vi "Test DUT Self Test Triggers Status Broadcast Message if Not Powered.vi"(8 "error in (no error)":errorcluster, 11 "Device Under Test Test In":refnum<class "Device Under Test Test.lvclass">) -> (0 "error out":errorcluster, 3 "Device Under Test Test Out":refnum<class "Device Under Test Test.lvclass">)   [LabVIEW 2020, in "Device Under Test Test.lvclass"]
uses:
  Device Under Test Test.lvclass
  C:/Program Files (x86)/National Instruments/LabVIEW 2020/vi.lib/Astemes/LUnit/Test Case.lvclass
  Device Under Test/Device Under Test.lvclass
  C:/Program Files (x86)/National Instruments/LabVIEW 2020/vi.lib/Astemes/Triarc Framework/Process/Process.lvclass
  <vilib>/Astemes/Triarc Framework/Process/Process.lvclass/Process.ctl
  <vilib>/Astemes/LUnit/Test Case.lvclass/Test Case.ctl
  <vilib>/Astemes/Triarc Framework/Broadcast Event Helpers/Execution timer.vi
  <vilib>/Astemes/Triarc Framework/Process/Private/SubVIs/Wait for finish.vi
  <vilib>/Astemes/Triarc Framework/Process/Private/SubVIs/Set Lifecycle State.vi
  <vilib>/Astemes/Triarc Framework/Process/Protected/Messaging/Send Message.vi
  <vilib>/Astemes/LUnit/Core/LUnit Test Case/Private/Append Pass Result.vi
  <vilib>/Astemes/LUnit/Core/LUnit Test Case/Private/Append Fail Result.vi
  <vilib>/Astemes/Triarc Framework/Process/Private/SubVIs/Handle Debug Data.vi
  <vilib>/Astemes/LUnit/Core/LUnit Test Case/Private/Run In UI.vi
  <vilib>/Utility/error.llb/Clear Errors.vi
  <vilib>/Astemes/Triarc Framework/Support/Dequeue Broadcast Message.vi
  <vilib>/Astemes/Triarc Framework/Process/Public/Lifecycle/Get Lifecycle State.vi
  <vilib>/Utility/error.llb/Error Cluster From Error Code.vi
  <vilib>/Astemes/Triarc Framework/Callback/Callback.lvclass
  <vilib>/Astemes/Triarc Framework/Process/Process.lvclass
  <vilib>/Astemes/LUnit/Test Case.lvclass
  <vilib>/Astemes/Triarc Framework/Broadcast Event Helpers/Broadcast Event Helpers.lvlib
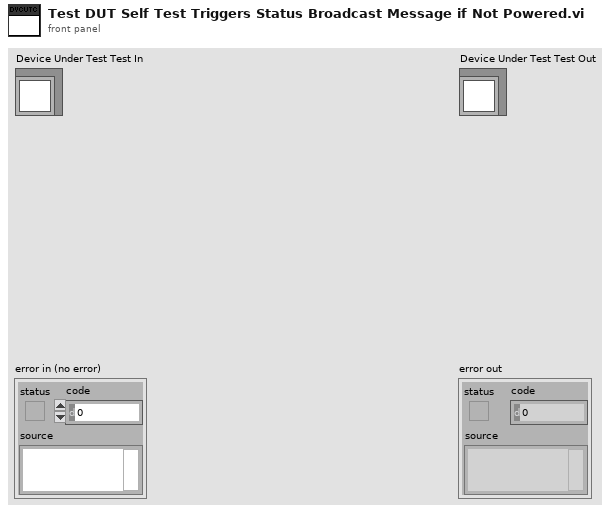
[diagram p1: front panel]
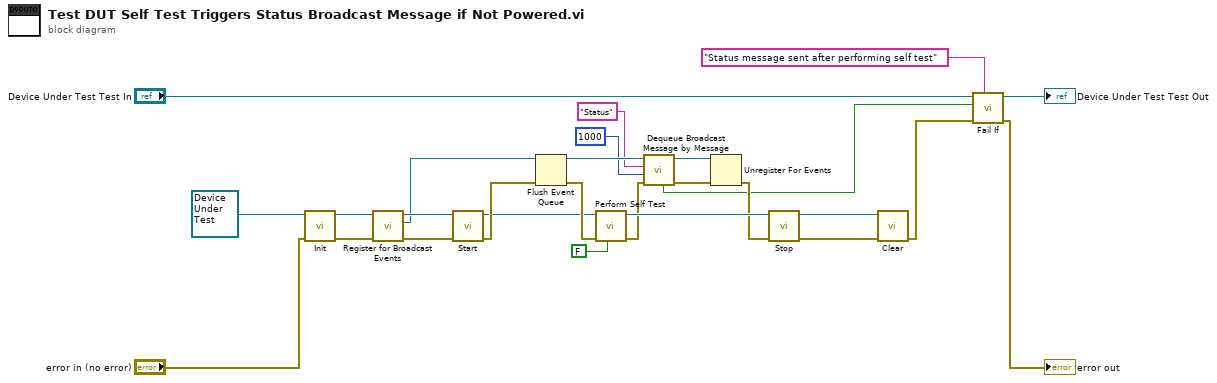
[diagram p0: block diagram]
diagram:
  n1 = call-dynamic "Init.vi"("error in (no error)"="error in (no error)", "View In"=refnum<class "Device Under Test.lvclass"> refnum ("Device Under Test.lvclass")) -> ("error out"=w19:errorcluster, "View Out"=w21:refnum<class "Device Under Test.lvclass">)  [unwired: 8 in]
  n2 = call <vilib>:"Register for Broadcast Events.vi"("error in (no error)"=w19, "Process In"=w21) -> ("error out"=w18:errorcluster, "Event Registration Refnum Out"=w8:refnum<event-registration>, "Process Out"=w20:refnum<class "Device Under Test.lvclass">)  [unwired: 7 in]
  n3 = call <vilib>:"Start.vi"("error in (no error)"=w18, "Process In"=w20) -> ("error out"=w26:errorcluster, "Process Out"=w2:refnum<class "Device Under Test.lvclass">)  [unwired: 7 in, 1 out]
  n4 = Flush Event Queue(0:w8, 3:w26) -> (8:w7:refnum<event-registration>, 11:w9:errorcluster)  [unwired: 4 in, 1 out]
  n5 = call "Perform Self Test.vi"("Wait for Reply?"=FALSE, "error in (no error)"=w9, "Device Under Test In"=w2) -> ("error out"=w11:errorcluster, "Device Under Test Out"=w25:refnum<class "Device Under Test.lvclass">)  [unwired: 5 in, 2 out]
  n6 = call <vilib>:"Dequeue Broadcast Message by Message.vi"("error in (no error)"=w11, "Timeout (-1)"=1000, "Message"="Status", "Event Registration Refnum"=w7) -> ("error out"=w10:errorcluster, "Event Registration Refnum Out"=w5:refnum<event-registration>, "Timed Out?"=w3:bool)  [unwired: 3 in, 2 out]
  n7 = Unregister For Events(event registration refnum=w5, error in=w10) -> (error out=w6:errorcluster)
  n8 = call <vilib>:"Stop.vi"("error in (no error)"=w6, "Process In"=w25) -> ("error out"=w23:errorcluster, "Process Out"=w24:refnum<class "Device Under Test.lvclass">)  [unwired: 7 in, 1 out]
  n9 = call-dynamic "Clear.vi"("error in (no error)"=w23, "View In"=w24) -> ("error out"=w16:errorcluster)  [unwired: 9 in]
  n10 = call <vilib>:"Fail If.vi"("Description"="Status message sent after performing self test", "error in (no error)"=w16, "Fail?"=w3, "LUnit Test Case In"="Device Under Test Test In") -> ("error out"=→"error out":errorcluster, "LUnit Test Case Out"=→"Device Under Test Test Out":refnum<class "Device Under Test Test.lvclass">)  [unwired: 6 in]
